vi "Close Instrument.vi"(8 "error in (no error)":errorcluster, 11 "VNA":refnum<class "VNA.lvclass">) -> (0 "error out":errorcluster, 3 "VNA out":refnum<class "VNA.lvclass">)   [LabVIEW 2016, in "VNA.lvclass"]
uses:
  VNA.lvclass
  P:/users1/Dengyu/Agilent 87XX Series/Agilent 87XX Series.lvlib
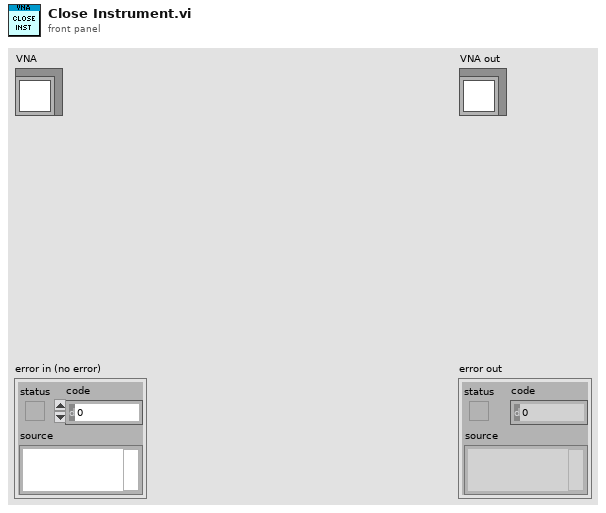
[diagram p1: front panel]
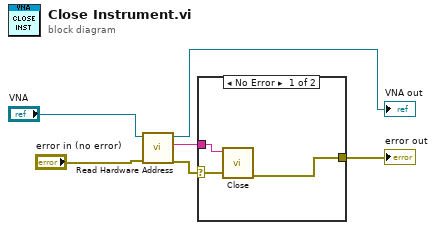
[diagram p0: block diagram]
diagram:
  n1 = call-dynamic "Read Hardware Address.vi"("error in (no error)"="error in (no error)", "Instrument in"="VNA") -> ("error out"=w1:errorcluster, "Hardware Address"=w2:string, "Instrument out"=→"VNA out":refnum<class "VNA.lvclass">)  [unwired: 7 in]
  n2 = case shown="No Error" w1 {
    selector: w1 -> [w8 w10]
    tunnel: [w9 w10] -> w3
    tunnel: w2 -> [w7 _]
    frame No Error {
      n3 = call "Close.vi"("error in (no error)"=w8, "VISA resource name"=w7) -> ("error out"=w9:errorcluster)  [unwired: 9 in]
    }
    frame Error {
    }
  }
  "error out" <- w3
